vi "Release ByRef (Unnamed SEQ).vi"(8 "error in (no error)":errorcluster, 11 "Numeric in":refnum<class "Numeric Test Object.lvclass">) -> (0 "error out":errorcluster, 3 "Numeric out":refnum<class "Numeric Test Object.lvclass">)   [LabVIEW 2009, in "Numeric Test Object.lvclass"]
doc: "Releases the unnamed queue used for by-ref data."
uses:
  Numeric Test Object.lvclass
  Numeric Test Object.lvclass/Numeric Test Object.ctl
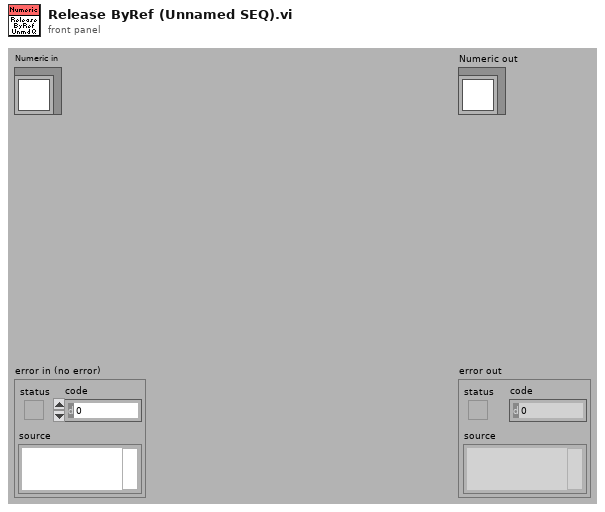
[diagram p1: front panel]
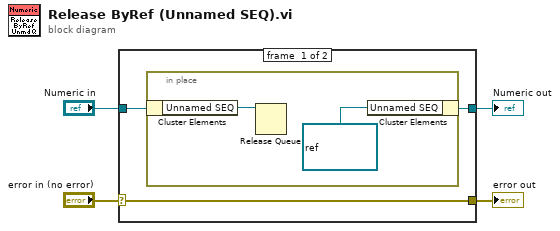
[diagram p0: block diagram]
diagram:
  n1 = case shown="No Error" "error in (no error)" {
    selector: "error in (no error)" -> [w7 w11]
    tunnel: [w7 w11] -> w3
    tunnel: [w5 w10] -> w1
    tunnel: "Numeric in" -> [w6 w10]
    frame #0 {
      n2 = in-place {
        n3 = in-place-cluster #1(w6) -> ("Unnamed SEQ"=w9:refnum<queue>)
        n4 = Release Queue(queue=w9) -> ()  [unwired: 2 in, 3 out]
        n5 = in-place-cluster #1("Unnamed SEQ"=refnum<queue> refnum) -> (w5:refnum<class "Numeric Test Object.lvclass">)
      }
    }
    frame #1 {
    }
  }
  "error out" <- w3
  "Numeric out" <- w1
